vi "PAN_FindComs.vi"(10 "comsmod":string="single_tcp", 11 "modules":path) -> (3 "coms to run":path[](array[path]))   [LabVIEW 2016]
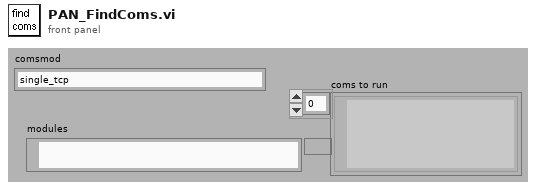
[diagram p1: front panel]
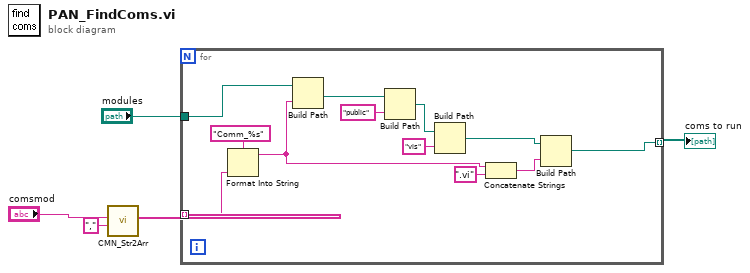
[diagram p0: block diagram]
diagram:
  n1 = call "CMN_Str2Arr.vi"("separator"=",", "string in"="comsmod") -> ("Array out"=w3:string[])  [unwired: 2 in, 7 out]
  n2 = for {
    tunnel: [w17] -> w5 mode=indexing
    tunnel: w3 -> [w9] mode=indexing
    tunnel: "modules" -> [w10]
    n3 = Format Into String(format string="Comm_%s", w9) -> (resulting string=w8:string)  [unwired: 2 in, 1 out]
    n4 = Build Path(base path=w10, name or relative path=w8) -> (appended path=w7:path)
    n5 = Build Path(base path=w7, name or relative path="public") -> (appended path=w12:path)
    n6 = Build Path(base path=w12, name or relative path="vis") -> (appended path=w6:path)
    n7 = Concatenate Strings(w8, ".vi" ("string")) -> (w14:string)
    n8 = Build Path(base path=w6, name or relative path=w14) -> (appended path=w17:path)
  }
  "coms to run" <- w5
